vi "7.0.0_Finalization_NG_unit.vi"(7 "Data in":T1, 8 "error in (no error)":errorcluster, 9 "AllControls In":T2, 10 "?":T3, 11 "Message Queue out":T4) -> (0 "error out":errorcluster, 1 "Flow":string, 2 "Data":T3, 3 "Message Queue Out":T4, 5 "Data out":T1)   [LabVIEW 2017]
uses:
  Depends/AMC/subVIs/TypeDefs/amc_Message Queue.ctl
  Depends/AMC/subVIs/TypeDefs/amc_Message.ctl
  Depends/Tools/Keyed Array/Tools_KeyedArray KeyedArray.ctl
  Ctrls/Data.ctl
  Ctrls/AllControls.ctl
  Ctrls/CSV_Data.ctl
  DIPC 692 Daemon API/typdef/device_mode.ctl
  DIPC 692 Daemon API/typdef/read_nvm_section.ctl
  Ctrls/PathChoose.ctl
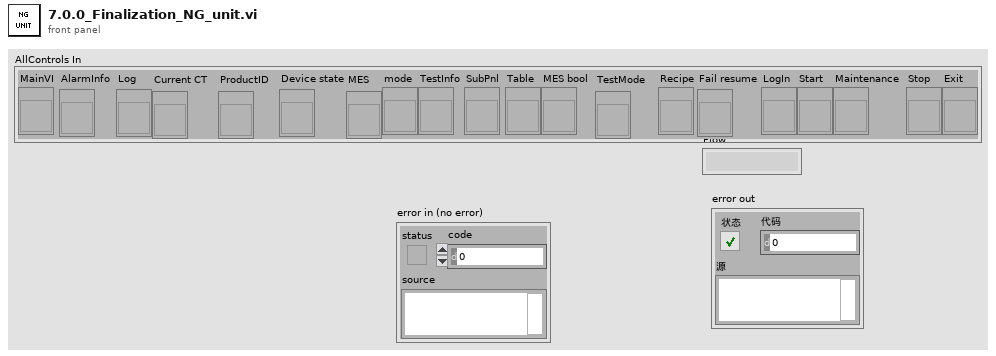
[diagram p1: front panel]
types:
  T1 = typedef "CSV_Data.ctl" = cluster{"Initialisation":cluster{"LMT - Connect UUT (con COM)":string, "LMT - Software Version (rrel)":string, "LMT - Write SKU file (wskuc)":string, "LMT - SKU file name":string, "Connect UUT DDM":string, "Read DDM EOL Timestamp - Mode":string, "Read DDM EOL Timestamp - Timestamp":string, "Read DDM EOL Timestamp - Rig ID":string, "Read DDM EOL Timestamp - Passmark ID":string, "Read DDM EOL Timestamp - Passmark Rev":string, "Software Version before flashing":string, "Read Hardware Serial":string, "UUT DDM SN":string, "Compare DDM SN with MES SN":string, "Backup PCBA Calibration EEPROM Response - CAL":string, "Flash Firmware Version":string, "Check SW Version":string, "Read DDM SW Version after flashing":string, "Set SKU Config":string, "Ready Status":string, "Set Device Mode to EOL":string, "DDM Parameter - Voltage":string, "DDM Parameter - Current":string, "DDM Parameter - Power":string, "DDM Parameter - Speed":string, "DDM Parameter - Pressure":string, "Tester Parameter - Voltage":string, "Tester Parameter - Current":string, "Tester Parameter - Power":string, "Tester Parameter - Ambient Pressure":string, "Tester Parameter - Ambient Temperature":string, "Calculated Parameter - DDM Pressure Corrected":string, "Calculated Parameter - DDM Real Power":string, "Calculated Parameter - Delta V":string}, "BEMF_Calibration":cluster{"Calibration Result - eol_cold_bemf_temp":string, "DDM Ambient Temp":string, "Restriction Plate Diameter":string, "Calibration Result - eol_bemf_mp_cold_coef_a":string, "Calibration Result - eol_bemf_mp_cold_coef_b":string, "Calibration Result - eol_bemf_mp_cold_coef_c":string, "Calibration Result - eol_bemf_lsi_cold_ref_coeffs":string, "Get - Calibration Result - eol_bemf_lsi_speed":string, "Get - Calibration Result - eol_bemf_lsi_integral_0":string, "Calibration Result - eol_bemf_lsi_integral_1":string, "Get - Calibration Result - eol_bemf_lsi_integral_2":string, "Get - Calibration Result - eol_cold_bemf":string, "Get - Calibration Result - eol_cold_bemf_fisf":string, "Finalise Calibration":string, "Compare -Calibration Result - eol_cold_bemf":string, "Compare -Calibration Result - eol_cold_bemf_fisf":string}, "ECO":cluster{"Reset Power Tune":string, "Reset BEMF FISF Calibration":string, "Restriction Plate Diameter":string, "ECO - Stabilisation Time":string, "ECO - DDM Parameter - Voltage":string, "ECO - DDM Parameter - Current":string, "ECO - DDM Parameter - Power":string, "ECO - DDM Parameter - Measured Power":string, "ECO - DDM Parameter - Speed":string, "ECO - DDM Parameter - Pressure":string, "ECO - Tester Parameter - Voltage":string, "ECO - Tester Parameter - Current":string, "ECO - Tester Parameter - Power":string, "ECO - Tester Parameter - Ambient Pressure":string, "ECO - Tester Parameter - Ambient Temperature":string, "ECO - Tester Parameter - Ambient Humidity":string, "ECO - Calculated Parameter - DDM Pressure Corrected":string, "ECO - Calculated Parameter - DDM Real Power":string, "ECO - Calculated Parameter - Delta V":string, "ECO - Calculated Parameter - Flowrate":string, "ECO - Calculated Parameter - Airwatt":string, "ECO - Formula":string, "PT ECO - Power Tune Mode Status":string}, "BOOST":cluster{"Restriction Plate Diameter":string, "BOOST - Stabilisation Time":string, "BOOST - DDM Parameter - Voltage":string, "BOOST - DDM Parameter - Current":string, "BOOST - DDM Parameter - Power":string, "BOOST - DDM Parameter - Measured Power":string, "BOOST - DDM Parameter - Speed":string, "BOOST - DDM Parameter - Pressure":string, "BOOST - Tester Parameter - Voltage":string, "BOOST - Tester Parameter - Current":string, "BOOST - Tester Parameter - Power":string, "BOOST - Tester Parameter - Ambient Pressure":string, "BOOST - Tester Parameter - Ambient Temperature":string, "BOOST - Tester Parameter - Ambient Humidity":string, "BOOST - Calculated Parameter - DDM Pressure Corrected":string, "BOOST - Calculated Parameter - DDM Real Power":string, "BOOST - Calculated Parameter - Delta V":string, "BOOST - Calculated Parameter - Flowrate":string, "BOOST - Calculated Parameter - Airwatt":string, "BOOST - Get AM Presence":string, "Air Muscle Turn Off Status":string, "BOOST - Air Muscle Calculated Parameter - Airwatt B":string, "BOOST - Air Muscle Calculate Airwatt Delta":string, "PT BOOST - Power Tune Mode Status":string, "Finalise Calibration":string, "ECO - Get AW Calibration value":string, "BOOST - Get AW Calibration value":string}, "MAX":cluster{"Restriction Plate Diameter":string, "MAX - Stabilisation Time":string, "Get Average Delta Tmag (LSIdelta_FISFdelta_LSItmag_FISFtmag_IIRtmag)":string, "Get Average Delta Tmag FISF":string, "MAX - DDM Parameter - Voltage":string, "MAX - DDM Parameter - Current":string, "MAX - DDM Parameter - Power":string, "MAX - DDM Parameter - Measured Power":string, "MAX - DDM Parameter - Speed":string, "MAX - DDM Parameter - Pressure":string, "MAX - Tester Parameter - Voltage":string, "MAX - Tester Parameter - Current":string, "MAX - Tester Parameter - Power":string, "MAX - Tester Parameter - Ambient Pressure":string, "MAX - Tester Parameter - Ambient Temperature":string, "MAX - Tester Parameter - Ambient Humidity":string, "MAX - Calculated Parameter - DDM Pressure Corrected":string, "MAX - Calculated Parameter - DDM Real Power":string, "MAX - Calculated Parameter - Delta V":string, "MAX - Calculated Parameter - Flowrate":string, "MAX - Calculated Parameter - Airwatt":string, "MAX_FISF_Check_Average_Delta_Tmag":string, "MAX - FISF - BEMF Finetune Result":string, "MAX tune - Delta P1":string, "MAX tune - Calculated Parameter - Airwatt":string, "Calculate Delta Airwatts - MAX finetune - Delta P2":string, "MAX finetune - DDM Parameter - Voltage":string, "MAX finetune - DDM Parameter - Current":string, "MAX finetune - DDM Parameter - Power":string, "MAX finetune - DDM Parameter - Measured Power":string, "MAX finetune - DDM Parameter - Speed":string, "MAX finetune - DDM Parameter - Pressure":string, "MAX finetune - Tester Parameter - Voltage":string, "MAX finetune - Tester Parameter - Current":string, "MAX finetune - Tester Parameter - Power":string, "MAX finetune - Tester Parameter - Ambient Pressure":string, "MAX finetune - Tester Parameter - Ambient Temperature":string, "MAX finetune - Tester Parameter - Ambient Humidity":string, "MAX finetune - Calculated Parameter - DDM Pressure Corrected":string, "MAX finetune - Calculated Parameter - DDM Real Power":string, "MAX finetune - Calculated Parameter - Delta V":string, "MAX finetune - Calculated Parameter - Flowrate":string, "MAX finetune - Calculated Parameter - Airwatt":string, "Check Derate Result":string, "Delta Tmag FISF":string, "Get Hot BEMF Result":string, "Calculate delta Pressure":string, "Finalise Calibration":string, "Calculate & Check Delta BEMF":string, "Delta P Airwatts Value":string}, "LL":cluster{"DDM Ambient Temp":string, "Restriction Plate Diameter":string, "LL - DDM Parameter - Voltage":string, "LL - DDM Parameter - Current":string, "LL - DDM Parameter - Power":string, "LL - DDM Parameter - Measured Power":string, "LL - DDM Parameter - Speed":string, "LL - DDM Parameter - Pressure":string, "LL - Tester Parameter - Voltage":string, "LL - Tester Parameter - Current":string, "LL - Tester Parameter - Power":string, "LL - DDM Real Power":string, "LL - Calibrate Task Detect LL":string}, "HL":cluster{"HL - DDM Parameter - Voltage":string, "HL - DDM Parameter - Current":string, "HL - DDM Parameter - Power":string, "HL - DDM Parameter - Measured Power":string, "HL - DDM Parameter - Speed":string, "HL - DDM Parameter - Pressure":string, "HL - Tester Parameter - Voltage":string, "HL - Tester Parameter - Current":string, "HL - Tester Parameter - Power":string, "HL - DDM Real Power":string, "HL - Calibrate Task Detect HL":string}, "LH":cluster{"Restriction Plate Diameter":string, "LH - DDM Parameter - Voltage":string, "LH - DDM Parameter - Current":string, "LH - DDM Parameter - Power":string, "LH - DDM Parameter - Measured Power":string, "LH - DDM Parameter - Speed":string, "LH - DDM Parameter - Pressure":string, "LH - Tester Parameter - Voltage":string, "LH - Tester Parameter - Current":string, "LH - Tester Parameter - Power":string, "LH - DDM Real Power":string, "LH - Calibrate Task Detect LH":string}, "HH":cluster{"HH - DDM Parameter - Voltage":string, "HH - DDM Parameter - Current":string, "HH - DDM Parameter - Power":string, "HH - DDM Parameter - Measured Power":string, "HH - DDM Parameter - Speed":string, "HH - DDM Parameter - Pressure":string, "HH - Tester Parameter - Voltage":string, "HH - Tester Parameter - Current":string, "HH - Tester Parameter - Power":string, "HH - DDM Real Power":string, "HH - Calibrate Task Detect HH":string}, "Inlet Blockage Calibration":cluster{"Inlet Blockage Calibration - DDM Parameter - Voltage":string, "Inlet Blockage Calibration - DDM Parameter - Current":string, "Inlet Blockage Calibration - DDM Parameter - Power":string, "Inlet Blockage Calibration - DDM Parameter - Measured Power":string, "Inlet Blockage Calibration - DDM Parameter - Speed":string, "Inlet Blockage Calibration - DDM Parameter - Pressure":string, "Inlet Blockage Calibration - Tester Parameter - Voltage":string, "Inlet Blockage Calibration - Tester Parameter - Current":string, "Inlet Blockage Calibration - Tester Parameter - Power":string, "Inlet Blockage Calibration - DDM Real Power":string, "Calibration Inlet Blockage_E":string, "Finalise Calibration":string, "Get Task Detect LL":string, "Get Task Detect HL":string, "Get Task Detect LH":string, "Get Task Detect HH":string, "Calibration Inlet Blockage":string, "Calibration eol cold bemf temp":string}, "GOOD":cluster{"GOOD UNIT - Clear EEPROM Error Log":string, "GOOD UNIT - Write Product Timestamp - Mode":string, "GOOD UNIT - Write Product Timestamp - Timestamp":string, "GOOD UNIT - Write Product Timestamp - Rig ID":string, "GOOD UNIT - Write Product Timestamp - Passmark ID":string, "GOOD UNIT - Write Product Timestamp - Passmark Rev":string, "GOOD UNIT - Set Device Mode to PROD":string, "GOOD UNIT - Backup PCBA Calibration EEPROM Response":string, "GOOD UNIT - Check Security Bit":string, "GOOD UNIT - Set Calibration Lock":string, "GOOD UNIT - Get_Calibration_Lock":string, "GOOD UNIT - Disconnect UUT":string}, "NG":cluster{"NG UNIT - Read NVM Error":string, "NG UNIT - Set Device Mode to FCT":string, "NG UNIT - Backup PCBA Calibration EEPROM Response - CAL":string, "NG UNIT - Backup PCBA Calibration EEPROM Response - ERROR":string, "NG UNIT - Backup PCBA Calibration EEPROM Response - USAGE":string, "NG UNIT - Disconnect UUT":string}, "SN":string, "Table":string[][], "Count":cluster{"Total":i32, "OK":i32, "NG":i32, "Yield":dbl}, "Start Time":timestamp, "daemon reference":refnum<k5>, "CT":dbl, "Config":string[][], "OK/NG":bool, "Station ID":string, "MES DDM SN":string, "MES PCBA SN":string, "Retest":string, "Lux":string, "Initialisation_Status":cluster{"LMT - Connect UUT (con COM)":string, "LMT - Software Version (rrel)":string, "LMT - Write SKU file (wskuc)":string, "LMT - SKU file name":string, "Connect UUT DDM":string, "Read DDM EOL Timestamp - Mode":string, "Read DDM EOL Timestamp - Timestamp":string, "Read DDM EOL Timestamp - Rig ID":string, "Read DDM EOL Timestamp - Passmark ID":string, "Read DDM EOL Timestamp - Passmark Rev":string, "Software Version before flashing":string, "Read Hardware Serial":string, "UUT DDM SN":string, "Compare DDM SN with MES SN":string, "Backup PCBA Calibration EEPROM Response - CAL":string, "Flash Firmware Version":string, "Check SW Version":string, "Read DDM SW Version after flashing":string, "Set SKU Config":string, "Ready Status":string, "Set Device Mode to EOL":string, "DDM Parameter - Voltage":string, "DDM Parameter - Current":string, "DDM Parameter - Power":string, "DDM Parameter - Speed":string, "DDM Parameter - Pressure":string, "Tester Parameter - Voltage":string, "Tester Parameter - Current":string, "Tester Parameter - Power":string, "Tester Parameter - Ambient Pressure":string, "Tester Parameter - Ambient Temperature":string, "Calculated Parameter - DDM Pressure Corrected":string, "Calculated Parameter - DDM Real Power":string, "Calculated Parameter - Delta V":string}, "BEMF_Calibration_Status":cluster{"Calibration Result - eol_cold_bemf_temp":string, "DDM Ambient Temp":string, "Restriction Plate Diameter":string, "Calibration Result - eol_bemf_mp_cold_coef_a":string, "Calibration Result - eol_bemf_mp_cold_coef_b":string, "Calibration Result - eol_bemf_mp_cold_coef_c":string, "Calibration Result - eol_bemf_lsi_cold_ref_coeffs":string, "Get - Calibration Result - eol_bemf_lsi_speed":string, "Get - Calibration Result - eol_bemf_lsi_integral_0":string, "Calibration Result - eol_bemf_lsi_integral_1":string, "Get - Calibration Result - eol_bemf_lsi_integral_2":string, "Get - Calibration Result - eol_cold_bemf":string, "Get - Calibration Result - eol_cold_bemf_fisf":string, "Finalise Calibration":string, "Compare -Calibration Result - eol_cold_bemf":string, "Compare -Calibration Result - eol_cold_bemf_fisf":string}, "ECO_Status":cluster{"Reset Power Tune":string, "Reset BEMF FISF Calibration":string, "Restriction Plate Diameter":string, "ECO - Stabilisation Time":string, "ECO - DDM Parameter - Voltage":string, "ECO - DDM Parameter - Current":string, "ECO - DDM Parameter - Power":string, "ECO - DDM Parameter - Measured Power":string, "ECO - DDM Parameter - Speed":string, "ECO - DDM Parameter - Pressure":string, "ECO - Tester Parameter - Voltage":string, "ECO - Tester Parameter - Current":string, "ECO - Tester Parameter - Power":string, "ECO - Tester Parameter - Ambient Pressure":string, "ECO - Tester Parameter - Ambient Temperature":string, "ECO - Tester Parameter - Ambient Humidity":string, "ECO - Calculated Parameter - DDM Pressure Corrected":string, "ECO - Calculated Parameter - DDM Real Power":string, "ECO - Calculated Parameter - Delta V":string, "ECO - Calculated Parameter - Flowrate":string, "ECO - Calculated Parameter - Airwatt":string, "ECO - Formula":string, "PT ECO - Power Tune Mode Status":string}, "BOOST_Status":cluster{"Restriction Plate Diameter":string, "BOOST - Stabilisation Time":string, "BOOST - DDM Parameter - Voltage":string, "BOOST - DDM Parameter - Current":string, "BOOST - DDM Parameter - Power":string, "BOOST - DDM Parameter - Measured Power":string, "BOOST - DDM Parameter - Speed":string, "BOOST - DDM Parameter - Pressure":string, "BOOST - Tester Parameter - Voltage":string, "BOOST - Tester Parameter - Current":string, "BOOST - Tester Parameter - Power":string, "BOOST - Tester Parameter - Ambient Pressure":string, "BOOST - Tester Parameter - Ambient Temperature":string, "BOOST - Tester Parameter - Ambient Humidity":string, "BOOST - Calculated Parameter - DDM Pressure Corrected":string, "BOOST - Calculated Parameter - DDM Real Power":string, "BOOST - Calculated Parameter - Delta V":string, "BOOST - Calculated Parameter - Flowrate":string, "BOOST - Calculated Parameter - Airwatt":string, "BOOST - Get AM Presence":string, "Air Muscle Turn Off Status":string, "BOOST - Air Muscle Calculated Parameter - Airwatt B":string, "BOOST - Air Muscle Calculate Airwatt Delta":string, "PT BOOST - Power Tune Mode Status":string, "Finalise Calibration":string, "ECO - Get AW Calibration value":string, "BOOST - Get AW Calibration value":string}, "MAX_Status":cluster{"Restriction Plate Diameter":string, "MAX - Stabilisation Time":string, "Get Average Delta Tmag (LSIdelta_FISFdelta_LSItmag_FISFtmag_IIRtmag)":string, "Get Average Delta Tmag FISF":string, "MAX - DDM Parameter - Voltage":string, "MAX - DDM Parameter - Current":string, "MAX - DDM Parameter - Power":string, "MAX - DDM Parameter - Measured Power":string, "MAX - DDM Parameter - Speed":string, "MAX - DDM Parameter - Pressure":string, "MAX - Tester Parameter - Voltage":string, "MAX - Tester Parameter - Current":string, "MAX - Tester Parameter - Power":string, "MAX - Tester Parameter - Ambient Pressure":string, "MAX - Tester Parameter - Ambient Temperature":string, "MAX - Tester Parameter - Ambient Humidity":string, "MAX - Calculated Parameter - DDM Pressure Corrected":string, "MAX - Calculated Parameter - DDM Real Power":string, "MAX - Calculated Parameter - Delta V":string, "MAX - Calculated Parameter - Flowrate":string, "MAX - Calculated Parameter - Airwatt":string, "MAX_FISF_Check_Average_Delta_Tmag":string, "MAX - FISF - BEMF Finetune Result":string, "MAX tune - Delta P1":string, "MAX tune - Calculated Parameter - Airwatt":string, "Calculate Delta Airwatts - MAX finetune - Delta P2":string, "MAX finetune - DDM Parameter - Voltage":string, "MAX finetune - DDM Parameter - Current":string, "MAX finetune - DDM Parameter - Power":string, "MAX finetune - DDM Parameter - Measured Power":string, "MAX finetune - DDM Parameter - Speed":string, "MAX finetune - DDM Parameter - Pressure":string, "MAX finetune - Tester Parameter - Voltage":string, "MAX finetune - Tester Parameter - Current":string, "MAX finetune - Tester Parameter - Power":string, "MAX finetune - Tester Parameter - Ambient Pressure":string, "MAX finetune - Tester Parameter - Ambient Temperature":string, "MAX finetune - Tester Parameter - Ambient Humidity":string, "MAX finetune - Calculated Parameter - DDM Pressure Corrected":string, "MAX finetune - Calculated Parameter - DDM Real Power":string, "MAX finetune - Calculated Parameter - Delta V":string, "MAX finetune - Calculated Parameter - Flowrate":string, "MAX finetune - Calculated Parameter - Airwatt":string, "Check Derate Result":string, "Delta Tmag FISF":string, "Get Hot BEMF Result":string, "Calculate delta Pressure":string, "Finalise Calibration":string, "Calculate & Check Delta BEMF":string, "Delta P Airwatts Value":string}, "LL_Status":cluster{"DDM Ambient Temp":string, "Restriction Plate Diameter":string, "LL - DDM Parameter - Voltage":string, "LL - DDM Parameter - Current":string, "LL - DDM Parameter - Power":string, "LL - DDM Parameter - Measured Power":string, "LL - DDM Parameter - Speed":string, "LL - DDM Parameter - Pressure":string, "LL - Tester Parameter - Voltage":string, "LL - Tester Parameter - Current":string, "LL - Tester Parameter - Power":string, "LL - DDM Real Power":string, "LL - Calibrate Task Detect LL":string}, "HL_Status":cluster{"HL - DDM Parameter - Voltage":string, "HL - DDM Parameter - Current":string, "HL - DDM Parameter - Power":string, "HL - DDM Parameter - Measured Power":string, "HL - DDM Parameter - Speed":string, "HL - DDM Parameter - Pressure":string, "HL - Tester Parameter - Voltage":string, "HL - Tester Parameter - Current":string, "HL - Tester Parameter - Power":string, "HL - DDM Real Power":string, "HL - Calibrate Task Detect HL":string}, "LH_Status":cluster{"Restriction Plate Diameter":string, "LH - DDM Parameter - Voltage":string, "LH - DDM Parameter - Current":string, "LH - DDM Parameter - Power":string, "LH - DDM Parameter - Measured Power":string, "LH - DDM Parameter - Speed":string, "LH - DDM Parameter - Pressure":string, "LH - Tester Parameter - Voltage":string, "LH - Tester Parameter - Current":string, "LH - Tester Parameter - Power":string, "LH - DDM Real Power":string, "LH - Calibrate Task Detect LH":string}, "HH_Status":cluster{"HH - DDM Parameter - Voltage":string, "HH - DDM Parameter - Current":string, "HH - DDM Parameter - Power":string, "HH - DDM Parameter - Measured Power":string, "HH - DDM Parameter - Speed":string, "HH - DDM Parameter - Pressure":string, "HH - Tester Parameter - Voltage":string, "HH - Tester Parameter - Current":string, "HH - Tester Parameter - Power":string, "HH - DDM Real Power":string, "HH - Calibrate Task Detect HH":string}, "Inlet Blockage Calibration_Status":cluster{"Inlet Blockage Calibration - DDM Parameter - Voltage":string, "Inlet Blockage Calibration - DDM Parameter - Current":string, "Inlet Blockage Calibration - DDM Parameter - Power":string, "Inlet Blockage Calibration - DDM Parameter - Measured Power":string, "Inlet Blockage Calibration - DDM Parameter - Speed":string, "Inlet Blockage Calibration - DDM Parameter - Pressure":string, "Inlet Blockage Calibration - Tester Parameter - Voltage":string, "Inlet Blockage Calibration - Tester Parameter - Current":string, "Inlet Blockage Calibration - Tester Parameter - Power":string, "Inlet Blockage Calibration - DDM Real Power":string, "Calibration Inlet Blockage_E":string, "Finalise Calibration":string, "Get Task Detect LL":string, "Get Task Detect HL":string, "Get Task Detect LH":string, "Get Task Detect HH":string, "Calibration Inlet Blockage":string, "Calibration eol cold bemf temp":string}, "GOOD_Status":cluster{"GOOD UNIT - Clear EEPROM Error Log":string, "GOOD UNIT - Write Product Timestamp - Mode":string, "GOOD UNIT - Write Product Timestamp - Timestamp":string, "GOOD UNIT - Write Product Timestamp - Rig ID":string, "GOOD UNIT - Write Product Timestamp - Passmark ID":string, "GOOD UNIT - Write Product Timestamp - Passmark Rev":string, "GOOD UNIT - Set Device Mode to PROD":string, "GOOD UNIT - Backup PCBA Calibration EEPROM Response":string, "GOOD UNIT - Check Security Bit":string, "GOOD UNIT - Set Calibration Lock":string, "GOOD UNIT - Get_Calibration_Lock":string, "GOOD UNIT - Disconnect UUT":string}, "NG_Status":cluster{"NG UNIT - Read NVM Error":string, "NG UNIT - Set Device Mode to FCT":string, "NG UNIT - Backup PCBA Calibration EEPROM Response - CAL":string, "NG UNIT - Backup PCBA Calibration EEPROM Response - ERROR":string, "NG UNIT - Backup PCBA Calibration EEPROM Response - USAGE":string, "NG UNIT - Disconnect UUT":string}, "SKU":string, "Plate_Diameter":string, "Alarm":string}
  T2 = typedef "AllControls.ctl" = cluster{"MainVI":refnum<vi>, "AlarmInfo":refnum<vi>, "Log":refnum<vi>, "Current CT":refnum<vi>, "ProductID":refnum<vi>, "Device state":refnum<vi>, "MES":refnum<vi>, "mode":refnum<vi>, "TestInfo":refnum<vi>, "SubPnl":refnum<vi>, "Table":refnum<vi>, "MES bool":refnum<vi>, "TestMode":refnum<vi>, "Recipe":refnum<vi>, "Fail resume":refnum<vi>, "LogIn":refnum<vi>, "Start":refnum<vi>, "Maintenance":refnum<vi>, "Stop":refnum<vi>, "Exit":refnum<vi>}
  T3 = typedef "Data.ctl" = cluster{"Initialisation":cluster{"DDM_Parameter":dbl[], "DDM_Parameter_status":bool[], "Get_Tester_Parameter":dbl[], "Get_Tester_Parameter_status":bool[], "Cal_Tester_Parameter":dbl[], "Cal_Tester_Parameter_status":bool[], "sw_version_before_status":bool, "sw_version_after_status":bool, "Set_SKU_Config_With_LMT_status":bool, "FCT_timestamp_status":bool, "LMT_Connect_to_UUT_status":bool}, "BEMF_Calibration":cluster{"Read_ambient_temperature":dbl, "Calibration_Vaule":dbl[], "Calibration_Vaule _B":dbl[], "Calibration_Vaule_status":bool[], "Calibration_Vaule_B_status":bool[]}, "ECO":cluster{"DDM_Parameter":dbl[], "DDM_Parameter_status":bool[], "Get_Tester_Parameter":dbl[], "Get_Tester_Parameter_status":bool[], "Cal_Tester_Parameter":dbl[], "Cal_Tester_Parameter_status":bool[], "DDM_Parameter_after_power_tune":dbl[], "Get_Tester_Parameter_after_power_tune":dbl[], "Cal_Tester_Parameter_after_power_tune":dbl[], "Cal_Tester_Parameter_after_power_tune_status":bool[], "Delta_P":dbl}, "BOOST":cluster{"DDM_Parameter":dbl[], "DDM_Parameter_status":bool[], "Get_Tester_Parameter":dbl[], "Get_Tester_Parameter_status":bool[], "Cal_Tester_Parameter":dbl[], "Cal_Tester_Parameter_status":bool[], "DDM_Parameter_after_power_tune":dbl[], "Get_Tester_Parameter_after_power_tune":dbl[], "Cal_Tester_Parameter_after_power_tune":dbl[], "Cal_Tester_Parameter_after_power_tune_status":bool[], "airwatts_am_off":dbl, "AW_Delta_(AM_on_and_off)":dbl, "AW_Delta_(AM_on_and_off)_Status":bool, "Delta_P":dbl}, "MAX":cluster{"Average_Tmag_Data":cluster{"LSI Delta in degC":dbl, "FISF Delta in degc":dbl, "LSI Tmag in degC":dbl, "Fisf Tmag in degC":dbl, "IIR Tmag in degC":dbl}, "DDM_Parameter":dbl[], "DDM_Parameter_status":bool[], "Get_Tester_Parameter":dbl[], "Get_Tester_Parameter_status":bool[], "Cal_Tester_Parameter":dbl[], "BEMF_Finetune":cluster{"eol_bemf_mp_cold_coef_c":dbl, "eol_cold_bemf_fisf_offset":dbl}, "AW_Tune":cluster{"delta_P1":dbl, "delta_P_Setting":dbl}, "DDM_Parameter_after_Airwatts_Tune":dbl[], "Get_Tester_Parameter_after_Airwatts_Tune":dbl[], "Cal_Tester_Parameter_after_Airwatts_Tune":dbl[], "DDM_Parameter_after_Airwatts_Finetune":dbl[], "Get_Tester_Parameter_after_Airwatts_Finetune":dbl[], "Cal_Tester_Parameter_after_Airwatts_Finetune":dbl[], "AW_Finetune":cluster{"delta_P2":dbl, "delta_P_Setting":dbl}, "Delta_Tmag_after_tune":cluster{"LSI Delta in degC":dbl, "FISF Delta in degc":dbl, "LSI Tmag in degC":dbl, "Fisf Tmag in degC":dbl, "IIR Tmag in degC":dbl}, "Hot Bemf in mV":dbl, "DDM_Pressure":dbl, "Delta_Pressure":dbl, " Cold Bemf in mV":dbl, " delta Bemf":dbl, " delta p":dbl, "Delta_Pressure_status":bool, " delta Bemf_status":bool, "LSI Delta in degC_status":bool, "FISF Delta in degc_status":bool, "Max_check_derate_status_status":bool, "Average_All_data":dbl[][], "Average_Tmag_Data_status":bool[], "Average_Tmag_Data_after_tune_status":bool[], "Cal_Tester_Parameter_status":bool[], "Cal_Tester_Parameter_status_after_Airwatts_Tune":bool[], "Cal_Tester_Parameter_status_after_Airwatts_FineTune":bool[]}, "Task_Detect_Calib":cluster{"LL":cluster{"DDM_Parameter":dbl[], "DDM_Parameter_status":bool[], "Get_Tester_Parameter":dbl[], "Get_Tester_Parameter_status":bool[], "Set_task_detect_A":dbl, "Set_task_detect_A_Status":bool}, "HL":cluster{"DDM_Parameter":dbl[], "DDM_Parameter_status":bool[], "Get_Tester_Parameter":dbl[], "Get_Tester_Parameter_status":bool[], "Set_task_detect_B":dbl, "Set_task_detect_B_Status":bool}, "LH":cluster{"DDM_Parameter":dbl[], "DDM_Parameter_status":bool[], "Get_Tester_Parameter":dbl[], "Get_Tester_Parameter_status":bool[], "Set_task_detect_C":dbl, "Set_task_detect_C_Status":bool}, "HH":cluster{"DDM_Parameter":dbl[], "DDM_Parameter_status":bool[], "Get_Tester_Parameter":dbl[], "Get_Tester_Parameter_status":bool[], "Set_task_detect_D":dbl, "Read_and_check_calibration_Status":bool[], "Set_task_detect_D_Status":bool}, "Get_eol_inlet_blockage_E":dbl, "Calib_vaule":cluster{"Get_task_detect_LL":dbl, "Get_task_detect_HL":dbl, "Get_task_detect_LH":dbl, "Get_task_detect_HH":dbl, "eol_inlet_blockage":dbl, "eol_code_bemf_temp":dbl}, "calibrated temp":dbl, "Inlet_Blockage_Calibration":cluster{"DDM_Parameter":dbl[], "DDM_Parameter_status":bool[], "Get_Tester_Parameter":dbl[], "Get_Tester_Parameter_status":bool[]}, "Get_eol_inlet_blockage_E_Status":bool}, "good":cluster{"Write_Product_TS":cluster{"TIMESTAMP":i64, "RIG_ID":i64, "PASSMARK_ID":i64, "PASSMARK_REV":i64}, "Read_Product_TS":cluster{"TIMESTAMP":i64, "RIG_ID":i64, "PASSMARK_ID":i64, "PASSMARK_REV":i64}, "Good_Check_Secuity_Bit_Stauts":bool}}
  T4 = typedef "amc_Message Queue.ctl" = refnum<queue>
  T5 = typedef "HD Config.ctl" = cluster{" PC":cluster{"PC Address":u8[], "PC Port":i32}, "FCO":cluster{"COM":refnum<visa-resource-name>, "Baudrate":u32}, "DC Power ":cluster{"COM":refnum<visa-resource-name>, "Baudrate":u32}, "PW3336":cluster{"COM":refnum<visa-resource-name>, "Baudrate":u32}, "Lefoo":cluster{"COM":refnum<visa-resource-name>, "Baudrate":u32}, "Tempt&Hum":cluster{"COM":refnum<visa-resource-name>, "Baudrate":u32}, "DIPC":cluster{"COM":refnum<visa-resource-name>}, "Daemon":cluster{"IP Address":string, "Port":u16, "Retry":u16}, "NFC":cluster{"COM":refnum<visa-resource-name>, "Baudrate":u32}, "Fail_resume_mode":bool, "GRR":bool}
  T6 = typedef "TesterInfo.ctl" = cluster{"Station Name":string, "Station Code":string, "ES NO.":string, "Tester ID":string, "PassMark Revision":string, "Rig ID":string, "Deamon_vision":string, "Project Name":string, "FFTesterPath":path, "Enable_User":bool, "Mode":enum16{"682"}, "MES":bool}
  T7 = typedef "device_mode.ctl" = enum16{"FCT", "EOL", "PROD"}
  T8 = typedef "PathChoose.ctl" = enum16{"OperatorLog", "AutoRunLog", "AlmLog", "TestData", "AllTestData", "backup_nvm", "backup_before_flashing"}
  T9 = enum16{"open", "replace", "create", "open or create", "replace or create", "replace or create with confirmation"}
  T10 = typedef "read_nvm_section.ctl" = enum16{"CAL", "ERROR", "USAGE"}
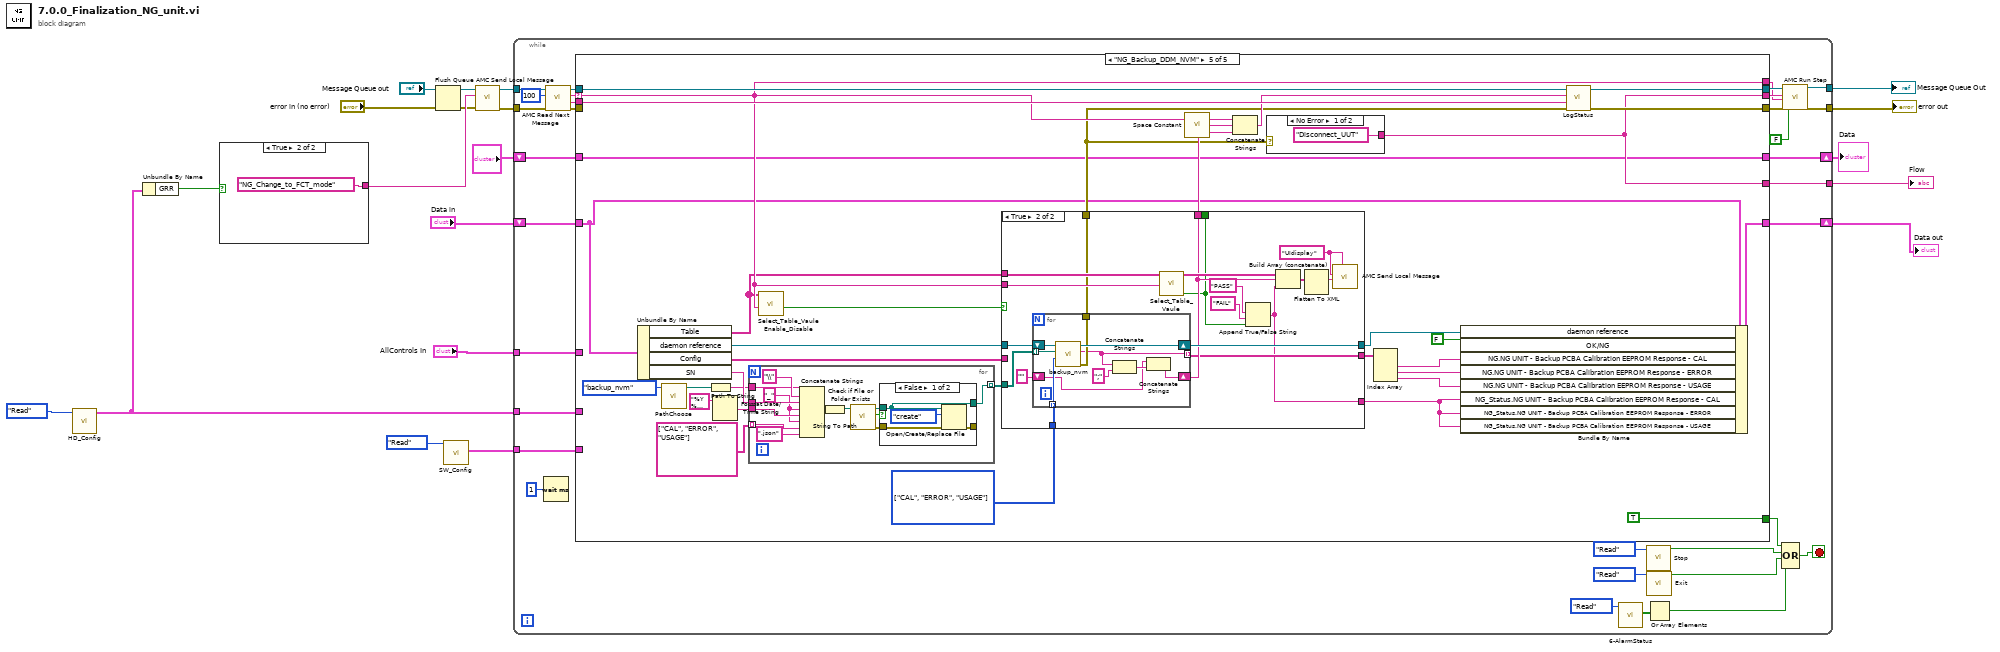
[diagram p0: block diagram]
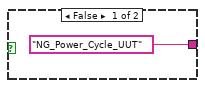
[diagram p2: hidden frame]
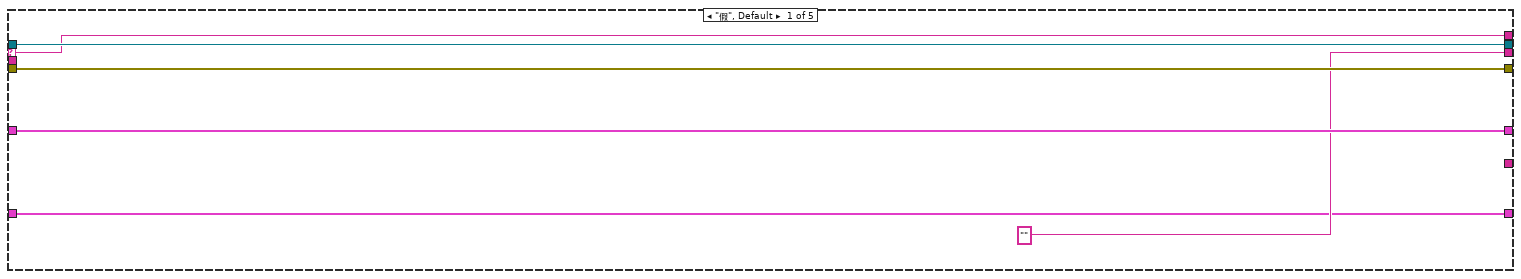
[diagram p3: hidden frame]
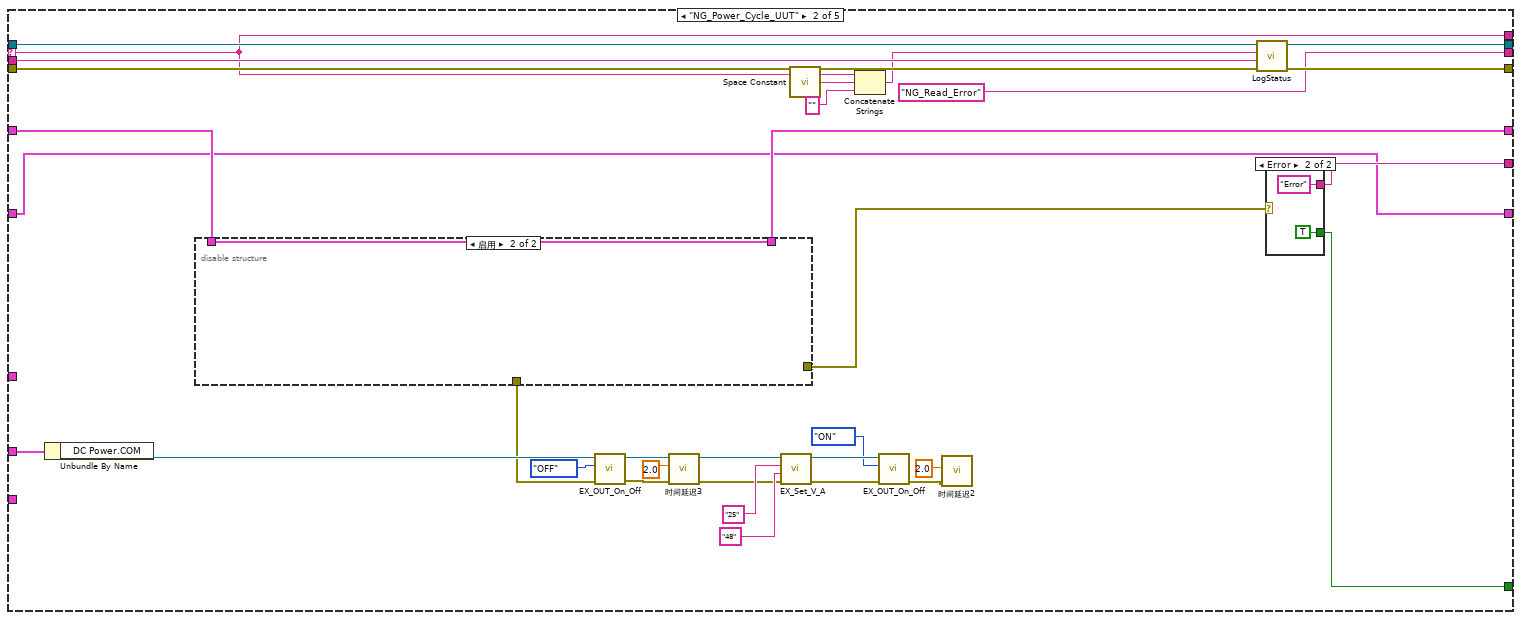
[diagram p4: hidden frame]
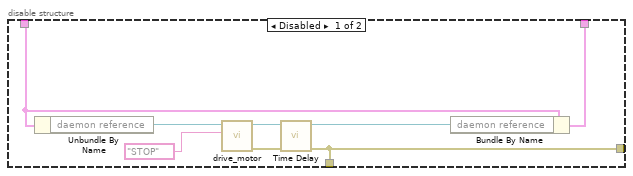
[diagram p5: hidden frame]
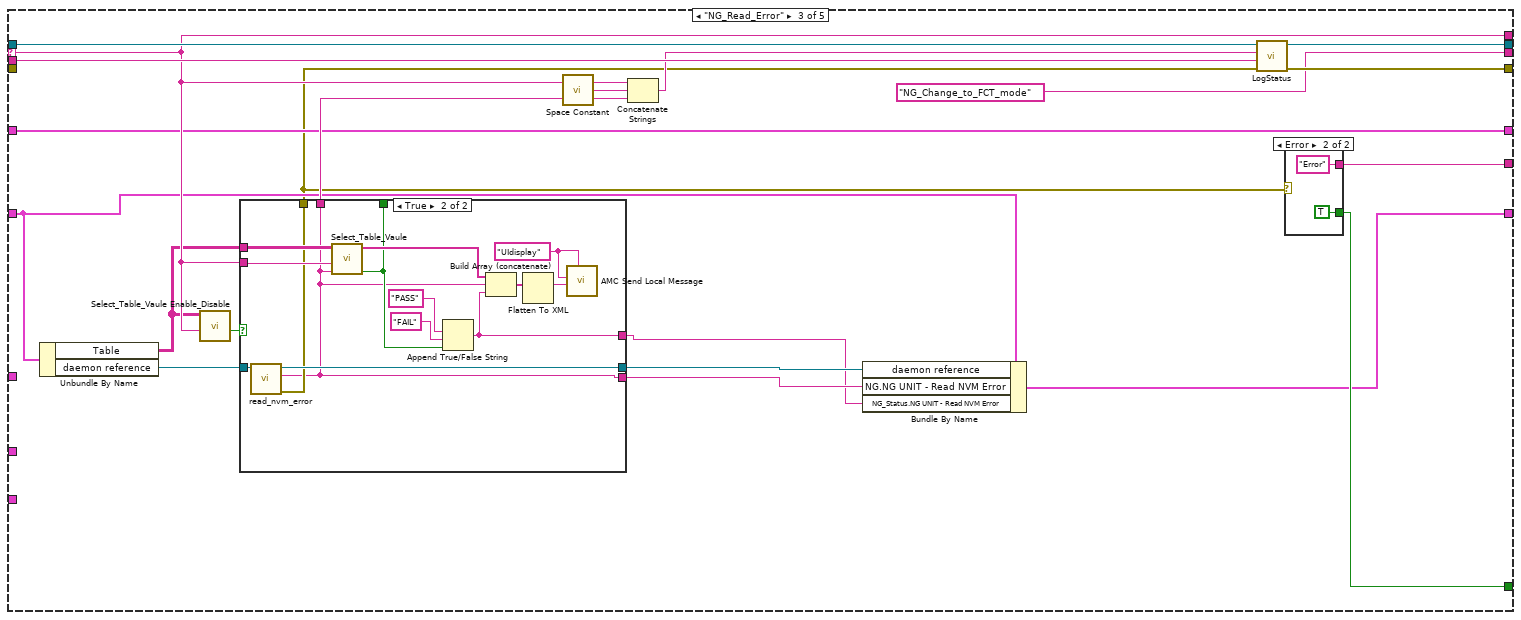
[diagram p7: hidden frame]
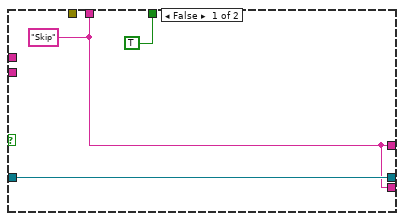
[diagram p9: hidden frame]
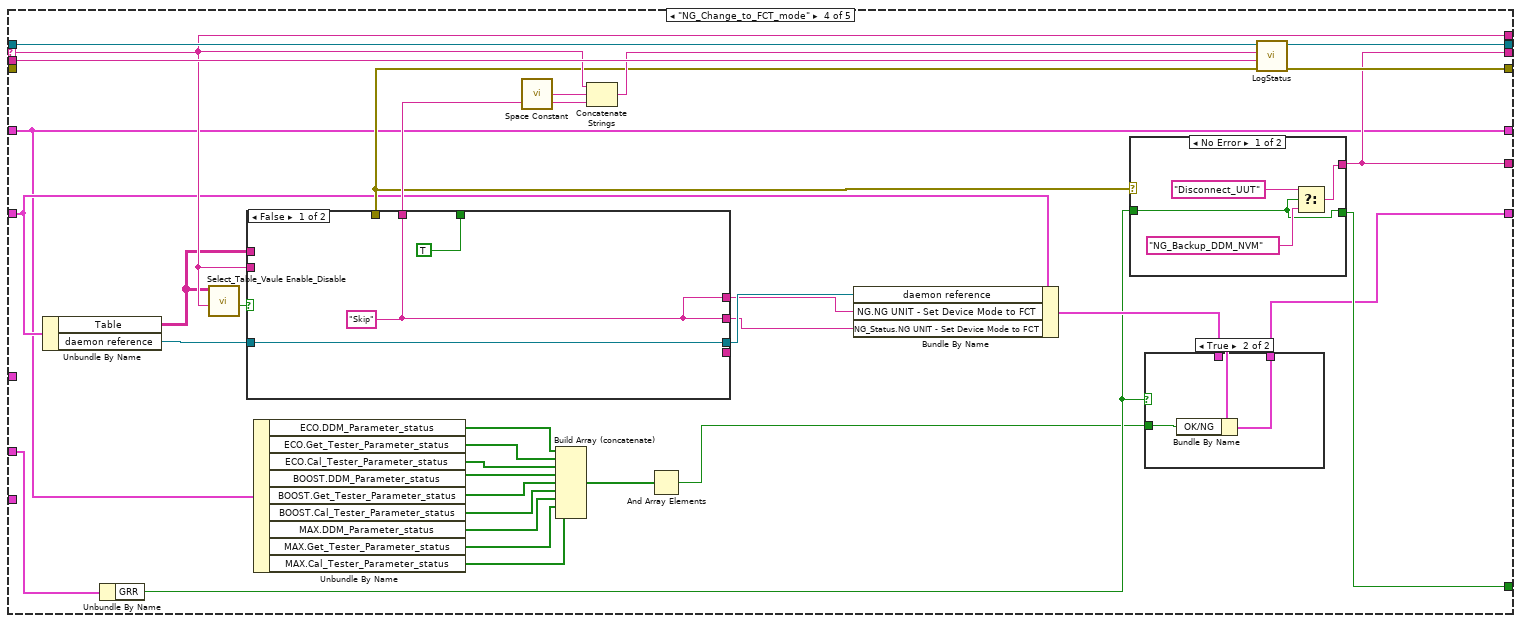
[diagram p10: hidden frame]
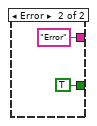
[diagram p12: hidden frame]
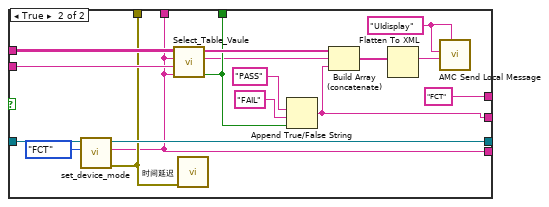
[diagram p13: hidden frame]
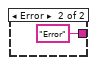
[diagram p14: hidden frame]
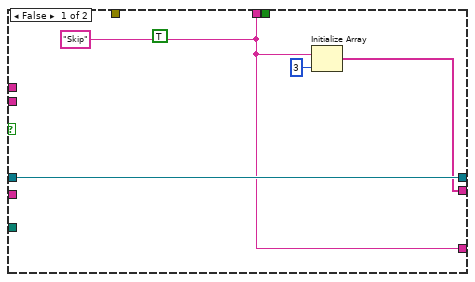
[diagram p16: hidden frame]
diagram:
  n1 = call "HD_Config.vi"("Step"=enum16{"Initial", "Write", "Read"}."Read") -> ("HD Config out"=w2:T5)  [unwired: 9 in, 1 out]
  n2 = Unbundle By Name(w2) -> ("GRR"=w1:bool)
  n3 = case shown="True" w1 {
    tunnel: ["NG_Power_Cycle_UUT" ("Message Name") "NG_Change_to_FCT_mode"] -> w18
    frame False {
    }
    frame True {
    }
  }
  n4 = Flush Queue(queue="Message Queue out") -> (queue out=w6:T4)  [unwired: 1 in, 2 out]
  n5 = call "SW_Config.vi"("Step"=enum16{"Initial", "Write", "Read"}."Read") -> ("SW Config out"=w9:T6)  [unwired: 9 in, 1 out]
  n6 = call "AMC Send Local Message.vi"("error in (no error)"="error in (no error)", "Message Name"=w18, "Message Queue in"=w6) -> ("error out"=w16:errorcluster, "Message Queue out"=w17:T4)  [unwired: 7 in]
  n7 = while {
    tunnel: w17 -> [w53]
    tunnel: [w49] -> w8
    tunnel: w16 -> [w47]
    tunnel: [w44] -> w7
    shift-right: [w40] -> w13
    shift-left: "?" -> [w41]
    tunnel: w2 -> [w39]
    tunnel: [w35] -> w11
    tunnel: w9 -> [w34]
    shift-right: [w25] -> w3
    shift-left: "Data in" -> [w27]
    tunnel: "AllControls In" -> [w26]
    stop <- w28 stop-if-true
    n8 = Wait (ms)(milliseconds to wait=u32 1 ("等待时间（毫秒）")) -> ()  [unwired: 1 out]
    n9 = call "AMC Read Next Message.vi"("error in (no error)"=w47, "timeout (1ms)"=100, "Message Queue in"=w53) -> ("error out"=w46:errorcluster, "Message Value"=w37:string, "Message Name"=w51:string, "Message Queue out"=w52:T4)  [unwired: 1 in, 4 out]
    n10 = case shown="\"NG_Backup_DDM_NVM\"" w51 {
      selector: w51 -> [w56 w83 w112 w164 w227]
      tunnel: w52 -> [w59 w89 w119 w171 w233]
      tunnel: [w59 w89 w119 w171 w233] -> w50
      tunnel: w46 -> [w58 w88 _ _ _]
      tunnel: [w58 w87 w118 w170 w232] -> w45
      tunnel: [_ w67 w108 w162 TRUE] -> w29
      tunnel: w41 -> [w57 w70 w106 w155 w206]
      tunnel: [w57 w69 w106 w155 w206] -> w40
      tunnel: w37 -> [_ w86 w117 w169 w231]
      tunnel: [w56 w83 w112 w164 w227] -> w36
      tunnel: w39 -> [_ w72 _ w156 _]
      tunnel: ["" "NG_Read_Error" "NG_Change_to_FCT_mode" w157 w216] -> w38
      tunnel: [_ w68 w109 w157 w216] -> w35
      tunnel: w34 -> [_ _ _ _ _]
      tunnel: w27 -> [w54 w64 w105 w159 w210]
      tunnel: w26 -> [_ _ _ _ _]
      tunnel: [w54 w64 w103 w144 w209] -> w25
      frame "假", Default {
      }
      frame "NG_Power_Cycle_UUT" {
        n11 = Unbundle By Name(w72) -> ("DC Power.COM"=w71:refnum<visa-resource-name>)
        n12 = disable-structure shown="启用" {
          disable-tunnel: w70 -> [w96 w97]
          disable-tunnel: [w95 w97] -> w69
          disable-tunnel: [w90 _] -> w66
          disable-tunnel: [w90 _] -> w65
          frame Disabled {
            n13 = Unbundle By Name(w96) -> ("daemon reference"=w92:refnum<k5>)
            n14 = call "drive_motor.vi"("Power Mode"="STOP", "daemon reference in"=w92) -> ("error out"=w93:errorcluster, "daemon reference out"=w94:refnum<k5>)  [unwired: 6 in, 2 out]
            n15 = call "Time Delay"("error in (no error)"=w93) -> ("error out"=w90:errorcluster)  [unwired: 10 in]
            n16 = Bundle By Name(cluster=w96, "daemon reference"=w94) -> (w95:T3)
          }
          frame Enabled {
          }
        }
        n17 = call "EX_OUT_On_Off.vi"("错误输入（无错误）"=w65, "Mode"=enum16{"ON", "OFF"}."OFF", "VISA resource name"=w71) -> ("error out"=w62:errorcluster, "VISA资源名称输出"=w75:refnum<visa-resource-name>)  [unwired: 7 in]
        n18 = call "时间延迟3"("error in (no error)"=w62, "Delay Time (s)"=2.0) -> ("error out"=w61:errorcluster)  [unwired: 9 in]
        n19 = call "EX_Set_V_A.vi"("错误输入（无错误）"=w61, "current"="48", "voltage"="25", "VISA resource name"=w75) -> ("error out"=w60:errorcluster, "VISA资源名称输出"=w78:refnum<visa-resource-name>)  [unwired: 6 in]
        n20 = call <vilib>:"Space Constant.vi"() -> ("String"=w85:string)
        n21 = Concatenate Strings(w83, w85, "" ("字符串")) -> (w84:string)
        n22 = call "EX_OUT_On_Off.vi"("错误输入（无错误）"=w60, "Mode"=enum16{"ON", "OFF"}."ON", "VISA resource name"=w78) -> ("error out"=w74:errorcluster)  [unwired: 7 in, 1 out]
        n23 = call "时间延迟2"("error in (no error)"=w74, "Delay Time (s)"=2.0) -> ()  [unwired: 9 in, 1 out]
        n24 = call "LogStatus.vi"("error in (no error)"=w88, "last message"=w86, "message"=w84) -> ("error  out"=w87:errorcluster)  [unwired: 8 in]
        n25 = case shown="Error" w66 {
          tunnel: [_ TRUE] -> w67
          tunnel: [_ "Error"] -> w68
          frame No Error {
          }
          frame Error {
          }
        }
      }
      frame "NG_Read_Error" {
        n26 = Unbundle By Name(w105) -> ("Table"=w111:string[][], "daemon reference"=w116:refnum<k5>)
        n27 = call "Select_Table_Vaule Enable_Disable.vi"("Action"=w112, "Table"=w111) -> ("Enable"=w113:bool)  [unwired: 8 in, 1 out]
        n28 = case shown="True" w113 {
          tunnel: w116 -> [w123 w138]
          tunnel: [TRUE w128] -> _
          tunnel: [w123 w132] -> w102
          tunnel: [w122 w126] -> w107
          tunnel: w112 -> [_ w131]
          tunnel: w111 -> [_ w130]
          tunnel: [_ w127] -> w104
          tunnel: [w122 w126] -> w101
          tunnel: [w122 w125] -> w100
          frame False {
            w122 = "Skip" ("response")
          }
          frame True {
            w137 = "UIdisplay" ("Process (\"\" - local)")
            n29 = call "read_nvm_error.vi"("daemon reference in"=w138) -> ("error out"=w127:errorcluster, "response"=w126:string, "daemon reference out"=w132:refnum<k5>)  [unwired: 7 in, 1 out]
            n30 = call "Select_Table_Vaule.vi"("Vaule"=w126, "Action"=w131, "Table"=w130) -> ("Result"=w128:bool, "vaule"=w129:string[])  [unwired: 7 in]
            n31 = Append True/False String(1:w128, 2:"FAIL" ("真字符串"), 3:"PASS" ("真字符串")) -> (0:w125:string)  [unwired: 1 in]
            n32 = Build Array (concatenate)(w129, w126, w125) -> (w136:string[])
            n33 = Flatten To XML(anything=w136) -> (xml string=w135:string)
            n34 = call "AMC Send Local Message.vi"("Process (\"\" - local)"=w137, "Message Value"=w135, "Message Name"=w137) -> ()  [unwired: 7 in, 2 out]
          }
        }
        n35 = call <vilib>:"Space Constant.vi"() -> ("String"=w115:string)
        n36 = Concatenate Strings(w112, w115, w107) -> (w114:string)
        n37 = Bundle By Name(cluster=w105, "daemon reference"=w102, "NG.NG UNIT - Read NVM Error"=w101, "NG_Status.NG UNIT - Read NVM Error"=w100) -> (w103:T1)
        n38 = call "LogStatus.vi"("error in (no error)"=w104, "last message"=w117, "message"=w114) -> ("error  out"=w118:errorcluster)  [unwired: 8 in]
        n39 = case shown="Error" w104 {
          tunnel: [_ TRUE] -> w108
          tunnel: [_ "Error"] -> w109
          frame No Error {
          }
          frame Error {
          }
        }
      }
      frame "NG_Change_to_FCT_mode" {
        n40 = Unbundle By Name(w159) -> ("Table"=w163:string[][], "daemon reference"=w168:refnum<k5>)
        n41 = Unbundle By Name(w156) -> ("GRR"=w143:bool)
        n42 = call "Select_Table_Vaule Enable_Disable.vi"("Action"=w164, "Table"=w163) -> ("Enable"=w165:bool)  [unwired: 8 in, 1 out]
        n43 = case shown="False" w165 {
          tunnel: w168 -> [w183 w195]
          tunnel: [TRUE w190] -> _
          tunnel: [w183 w194] -> w158
          tunnel: [w182 w187] -> w161
          tunnel: w164 -> [_ w193]
          tunnel: w163 -> [_ w192]
          tunnel: [_ w188] -> w160
          tunnel: [_ w187] -> _
          tunnel: [w182 w186] -> w140
          tunnel: [w182 "FCT" ("NG.NG UNIT - Set Device Mode to FCT")] -> w139
          frame False {
            w182 = "Skip" ("software string")
          }
          frame True {
            w200 = "UIdisplay" ("Process (\"\" - local)")
            n44 = call "set_device_mode.vi"("Mode"=device_mode."FCT", "daemon reference in"=w195) -> ("error out"=w188:errorcluster, "response"=w187:string, "daemon reference out"=w194:refnum<k5>)  [unwired: 6 in, 1 out]
            n45 = call "Select_Table_Vaule.vi"("Vaule"=w187, "Action"=w193, "Table"=w192) -> ("Result"=w190:bool, "vaule"=w191:string[])  [unwired: 7 in]
            n46 = call "时间延迟"("error in (no error)"=w188) -> ()  [unwired: 10 in, 1 out]
            n47 = Append True/False String(1:w190, 2:"FAIL" ("真字符串"), 3:"PASS" ("真字符串")) -> (0:w186:string)  [unwired: 1 in]
            n48 = Build Array (concatenate)(w191, w187, w186) -> (w199:string[])
            n49 = Flatten To XML(anything=w199) -> (xml string=w198:string)
            n50 = call "AMC Send Local Message.vi"("Process (\"\" - local)"=w200, "Message Value"=w198, "Message Name"=w200) -> ()  [unwired: 7 in, 2 out]
          }
        }
        n51 = Unbundle By Name(w155) -> ("ECO.DDM_Parameter_status"=w154:bool[], "ECO.Get_Tester_Parameter_status"=w153:bool[], "ECO.Cal_Tester_Parameter_status"=w152:bool[], "BOOST.DDM_Parameter_status"=w151:bool[], "BOOST.Get_Tester_Parameter_status"=w150:bool[], "BOOST.Cal_Tester_Parameter_status"=w149:bool[], "MAX.DDM_Parameter_status"=w148:bool[], "MAX.Get_Tester_Parameter_status"=w147:bool[], "MAX.Cal_Tester_Parameter_status"=w146:bool[])
        n52 = call <vilib>:"Space Constant.vi"() -> ("String"=w167:string)
        n53 = Build Array (concatenate)(w154, w153, w152, w151, w150, w149, w148, w147, w146) -> (w141:bool[])
        n54 = Concatenate Strings(w164, w167, w161) -> (w166:string)
        n55 = And Array Elements(Boolean array=w141) -> (logical AND=w142:bool)
        n56 = Bundle By Name(cluster=w159, "daemon reference"=w158, "NG.NG UNIT - Set Device Mode to FCT"=w139, "NG_Status.NG UNIT - Set Device Mode to FCT"=w140) -> (w145:T1)
        n57 = case shown="No Error" w160 {
          tunnel: [w176 TRUE] -> w162
          tunnel: [w177 "Error"] -> w157
          tunnel: w143 -> [w176 _]
          frame No Error {
            n58 = Select(t="Disconnect_UUT", s=w176, f="NG_Backup_DDM_NVM") -> (s? t:f=w177:string)
          }
          frame Error {
          }
        }
        n59 = case shown="True" w143 {
          tunnel: w145 -> [w172 w175]
          tunnel: [w172 w174] -> w144
          tunnel: w142 -> [_ w173]
          frame False {
          }
          frame True {
            n60 = Bundle By Name(cluster=w175, "OK/NG"=w173) -> (w174:T1)
          }
        }
        n61 = call "LogStatus.vi"("error in (no error)"=w160, "last message"=w169, "message"=w166) -> ("error  out"=w170:errorcluster)  [unwired: 8 in]
      }
      frame "NG_Backup_DDM_NVM" {
        w218 = T10[] [enum."CAL", enum."ERROR", enum."USAGE"] items=["CAL", "ERROR", "USAGE"]
        n62 = Unbundle By Name(w210) -> ("Table"=w226:string[][], "daemon reference"=w230:refnum<k5>, "Config"=w224:string[][], "SN"=w222:string)
        n63 = call "PathChoose.vi"(11:PathChoose."backup_nvm") -> ("Path_Out"=w213:path)  [unwired: 10 in]
        n64 = Path To String(path=w213) -> (string=w215:string)
        n65 = Format Date/Time String(time format string (%c)="%Y%m%d%H%M%S" ("时间格式字符串(%c)")) -> (date/time string=w221:string)  [unwired: 2 in]
        n66 = for {
          tunnel: w222 -> [w248]
          tunnel: w221 -> [w247]
          tunnel: string[] ["CAL", "ERROR", "USAGE"] -> [w245] mode=indexing
          tunnel: [w236] -> w219 mode=indexing
          tunnel: w215 -> [w242]
          w241 = "_" ("string")
          n67 = Concatenate Strings(w242, "\\" ("字符串"), w248, w241, w247, w241, w245, ".json" ("string")) -> (w246:string)
          n68 = String To Path(string=w246) -> (path=w237:path)
          n69 = call <vilib>:"Check if File or Folder Exists.vi"("path"=w237) -> ("error out"=w239:errorcluster, "file or folder exists?"=w240:bool, "dup path"=w238:path)  [unwired: 8 in]
          n70 = case shown="False" w240 {
            tunnel: w239 -> [w252 w253]
            tunnel: w238 -> [w249 w254]
            tunnel: [w249 w254] -> w236
            tunnel: [w251 w253] -> _
            frame False {
              n71 = Open/Create/Replace File(file path (use dialog)=w249, error in=w252, operation (0:open)=T9."create") -> (error out=w251:errorcluster)  [unwired: 3 in, 2 out]
            }
            frame True {
            }
          }
        }
        n72 = call "Select_Table_Vaule Enable_Disable.vi"("Action"=w227, "Table"=w226) -> ("Enable"=w225:bool)  [unwired: 8 in, 1 out]
        n73 = case shown="True" w225 {
          tunnel: w230 -> [w258 w271]
          tunnel: [w258 w270] -> w207
          tunnel: [w257 w266] -> w212
          tunnel: w227 -> [_ w269]
          tunnel: w226 -> [_ w268]
          tunnel: w224 -> [_ _]
          tunnel: [_ w265] -> _
          tunnel: w219 -> [_ w264]
          tunnel: w218 -> [_ w263]
          tunnel: [_ w261] -> w211
          tunnel: [w256 w260] -> w208
          tunnel: [w257 w259] -> w201
          frame False {
            w257 = "Skip" ("software string")
            (unwired) TRUE
            n74 = Initialize Array(w257, 3 ("维数大小")) -> (w256:string[])
          }
          frame True {
            w276 = "UIdisplay" ("Process (\"\" - local)")
            n75 = for {
              tunnel: w264 -> [w284] mode=indexing
              shift-right: [w285] -> w270
              shift-left: w271 -> [w286]
              tunnel: w263 -> [w283] mode=indexing
              shift-right: [w280] -> w266
              shift-left: "" -> [w279]
              tunnel: [w278] -> w261
              tunnel: [w277] -> w260 mode=indexing
              n76 = call "backup_nvm.vi"("type"=w283, "File Path"=w284, "daemon reference in"=w286) -> ("error out"=w278:errorcluster, "response"=w277:string, "daemon reference out"=w285:refnum<k5>)  [unwired: 5 in, 1 out]
              n77 = Concatenate Strings(w277, ";" ("字符串")) -> (w281:string)
              n78 = Concatenate Strings(w279, w281) -> (w280:string)
            }
            n79 = call "Select_Table_Vaule.vi"("Action"=w269, "Table"=w268) -> ("Result"=w265:bool, "vaule"=w267:string[])  [unwired: 8 in]
            n80 = Append True/False String(1:w265, 2:"FAIL" ("真字符串"), 3:"PASS" ("真字符串")) -> (0:w259:string)  [unwired: 1 in]
            n81 = Build Array (concatenate)(w267, w266, w259) -> (w275:string[])
            n82 = Flatten To XML(anything=w275) -> (xml string=w274:string)
            n83 = call "AMC Send Local Message.vi"("Process (\"\" - local)"=w276, "Message Value"=w274, "Message Name"=w276) -> ()  [unwired: 7 in, 2 out]
          }
        }
        n84 = call <vilib>:"Space Constant.vi"() -> ("String"=w229:string)
        n85 = Concatenate Strings(w227, w229, w212) -> (w228:string)
        n86 = case shown="No Error" w211 {
          tunnel: ["Disconnect_UUT" "Error"] -> w216
          frame No Error {
          }
          frame Error {
          }
        }
        n87 = Index Array(array=w208) -> (element #1=w204:string, element #2=w203:string, element #3=w202:string)  [unwired: 3 in]
        n88 = Bundle By Name(cluster=w210, "daemon reference"=w207, "OK/NG"=FALSE, "NG.NG UNIT - Backup PCBA Calibration EEPROM Response - CAL"=w204, "NG.NG UNIT - Backup PCBA Calibration EEPROM Response - ERROR"=w203, "NG.NG UNIT - Backup PCBA Calibration EEPROM Response - USAGE"=w202, "NG_Status.NG UNIT - Backup PCBA Calibration EEPROM Response - CAL"=w201, "NG_Status.NG UNIT - Backup PCBA Calibration EEPROM Response - ERROR"=w201, "NG_Status.NG UNIT - Backup PCBA Calibration EEPROM Response - USAGE"=w201) -> (w209:T1)
        n89 = call "LogStatus.vi"("error in (no error)"=w211, "last message"=w231, "message"=w228) -> ("error  out"=w232:errorcluster)  [unwired: 8 in]
      }
    }
    n90 = call "6-AlarmStatus.vi"("Step"=enum16{"Initial", "Write", "Read"}."Read") -> ("AlarmValue Out"=w23:bool[])  [unwired: 9 in, 1 out]
    n91 = call "Stop.vi"("Step"=enum16{"Initial", "Write", "Read"}."Read") -> ("Stop Out"=w31:bool)  [unwired: 9 in, 1 out]
    n92 = call "Exit.vi"("Step"=enum16{"Initial", "Write", "Read"}."Read" ("step")) -> ("Exit Out"=w30:bool)  [unwired: 9 in, 1 out]
    n93 = Or Array Elements(Boolean array=w23) -> (logical OR=w22:bool)
    n94 = Compound Arithmetic op=OR(w29, w31, w30, w22) -> (w28:bool)
    n95 = call "AMC Run Step.vi"("Message Queue In"=w50, "Message Name"=w38, "Message Value"=w36, "error in (no error)"=w45, "Mli/Sig"=FALSE) -> ("Message Queue Out"=w49:T4, "error out"=w44:errorcluster)  [unwired: 13 in]
  }
  "Message Queue Out" <- w8
  "error out" <- w7
  "Data" <- w13
  "Flow" <- w11
  "Data out" <- w3
